vi "Station - Search Serial Number by Device Name.vi"(6 "Ref?":bool=TRUE, 8 "error in (no error)":errorcluster, 10 "Data":string[](array[string]), 11 "Array in":refnum<vi>[](array[refnum])) -> (0 "error out":errorcluster, 1 "Channel":i32[](array[numeric]), 2 "Index":i32[](array[numeric]), 3 "IP Address":string[](array[string]))   [LabVIEW 2019]
uses:
  Controls/Global - IP Address.vi
  Controls/Global - Device.vi
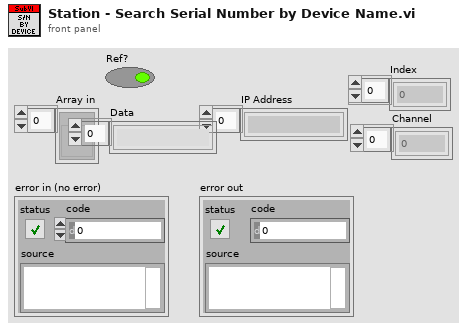
[diagram p1: front panel]
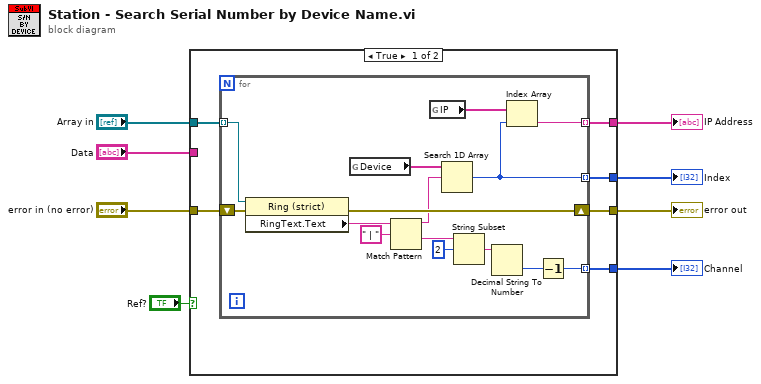
[diagram p0: block diagram]
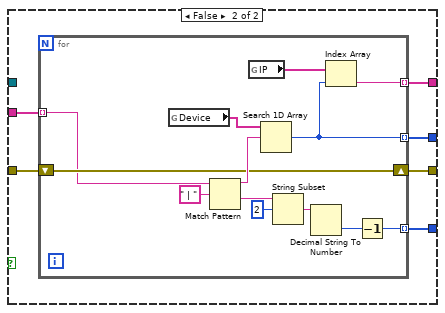
[diagram p2: hidden frame]
diagram:
  n1 = case shown="True" "Ref?" {
    tunnel: "Array in" -> [w14 _]
    tunnel: "error in (no error)" -> [w13 w35]
    tunnel: [w12 w34] -> w6
    tunnel: [w11 w33] -> w5
    tunnel: [w10 w32] -> w4
    tunnel: [w9 w31] -> w3
    tunnel: "Data" -> [_ w30]
    frame True {
      n2 = for {
        shift-right: [w27] -> w12
        shift-left: w13 -> [w29]
        tunnel: w14 -> [w28] mode=indexing
        tunnel: [w26] -> w11 mode=indexing
        tunnel: [w25] -> w10 mode=indexing
        tunnel: [w15] -> w9 mode=indexing
        n3 = property class="Ring (strict)"(reference=w28, error in=w29) -> (error out=w27:errorcluster, "RingText.Text"=w22:string)  [unwired: 1 out]
        n4 = global read "Global - Device.vi" "Device"() -> (w23:string[])
        n5 = Match Pattern(string=w22, regular expression=" | ") -> (before substring=w20:string, after substring=w17:string)  [unwired: 1 in, 2 out]
        n6 = global read "Global - IP Address.vi" "IP"() -> (w24:string[])
        n7 = Search 1D Array(1D array=w23, element=w20) -> (index of element=w25:i32)  [unwired: 1 in]
        n8 = String Subset(string=w17, offset (0)=2) -> (substring=w19:string)  [unwired: 1 in]
        n9 = Decimal String To Number(string=w19) -> (number=w16:i32)  [unwired: 2 in, 1 out]
        n10 = Index Array(array=w24, index=w25) -> (element=w26:string)
        n11 = Decrement(x=w16) -> (x-1=w15:i32)
      }
    }
    frame False {
      n12 = for {
        shift-right: [w37] -> w34
        shift-left: w35 -> [w37]
        tunnel: [w48] -> w33 mode=indexing
        tunnel: [w47] -> w32 mode=indexing
        tunnel: [w38] -> w31 mode=indexing
        tunnel: w30 -> [w36] mode=indexing
        n13 = global read "Global - Device.vi" "Device"() -> (w45:string[])
        n14 = Match Pattern(string=w36, regular expression=" | ") -> (before substring=w43:string, after substring=w40:string)  [unwired: 1 in, 2 out]
        n15 = global read "Global - IP Address.vi" "IP"() -> (w46:string[])
        n16 = Search 1D Array(1D array=w45, element=w43) -> (index of element=w47:i32)  [unwired: 1 in]
        n17 = String Subset(string=w40, offset (0)=2) -> (substring=w42:string)  [unwired: 1 in]
        n18 = Decimal String To Number(string=w42) -> (number=w39:i32)  [unwired: 2 in, 1 out]
        n19 = Index Array(array=w46, index=w47) -> (element=w48:string)
        n20 = Decrement(x=w39) -> (x-1=w38:i32)
      }
    }
  }
  "error out" <- w6
  "IP Address" <- w5
  "Index" <- w4
  "Channel" <- w3
